vi "Acquire.vi"(8 "error in (no error)":errorcluster, 10 "Message Queues":T1, 11 "Hardware Resources in":T4) -> (0 "error out":errorcluster, 2 "Message Queues out":T1, 3 "Hardware Resources out":T4)   [LabVIEW 2019, in "Acquisition.lvlib"]
doc: "Perform the acquisition. Replace the contents of this diagram with calls to acquisition hardware."
uses:
  Acquisition.lvlib
  Hardware Configuration.ctl
  Signal Type.ctl
  Support/Message Queue/All Message Queues.ctl
  Support/Message Queue/Message Cluster.ctl
  Controls/Data Queue.ctl
  Controls/Acquired Data.ctl
  Controls/Data Notifier.ctl
  Support/Message Queue/Message Queue.lvlib
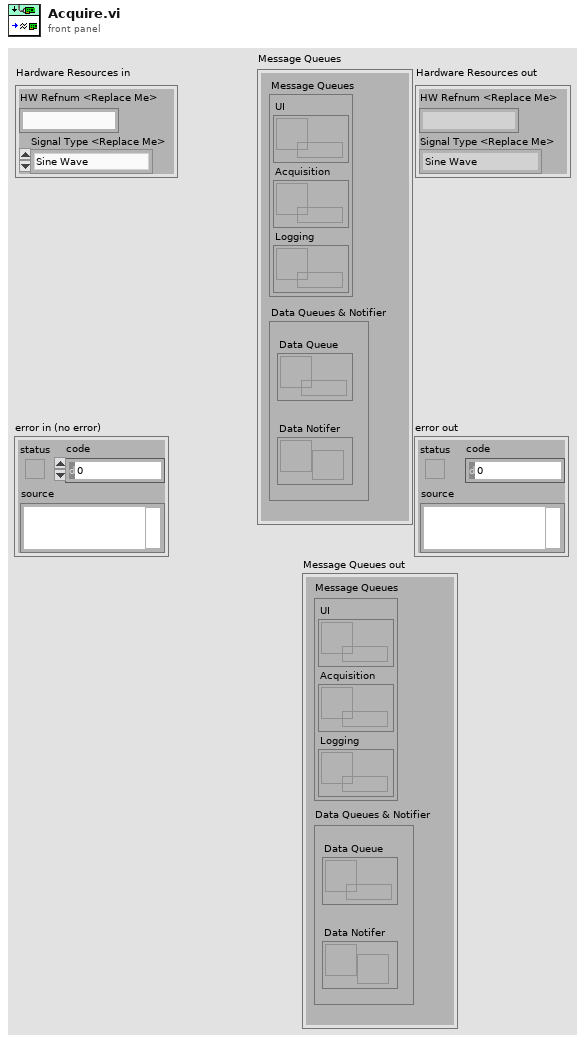
[diagram p1: front panel]
types:
  T1 = typedef "Message Queue.lvlib/All Message Queues.ctl" = cluster{"Message Queues":cluster{"UI":refnum<queue>, "Acquisition":refnum<queue>, "Logging":refnum<queue>}, "Data Queues & Notifier":cluster{"Data Queue":T2, "Data Notifer":T3}}
  T2 = typedef "Data Queue.ctl" = refnum<queue>
  T3 = typedef "Data Notifier.ctl" = refnum<notifier>
  T4 = typedef "Acquisition.lvlib/Hardware Configuration.ctl" = cluster{"HW Refnum <Replace Me>":string, "Signal Type <Replace Me>":T5}
  T5 = typedef "Acquisition.lvlib/Signal Type.ctl" = enum16{"Sine Wave", "Square with Noise"}
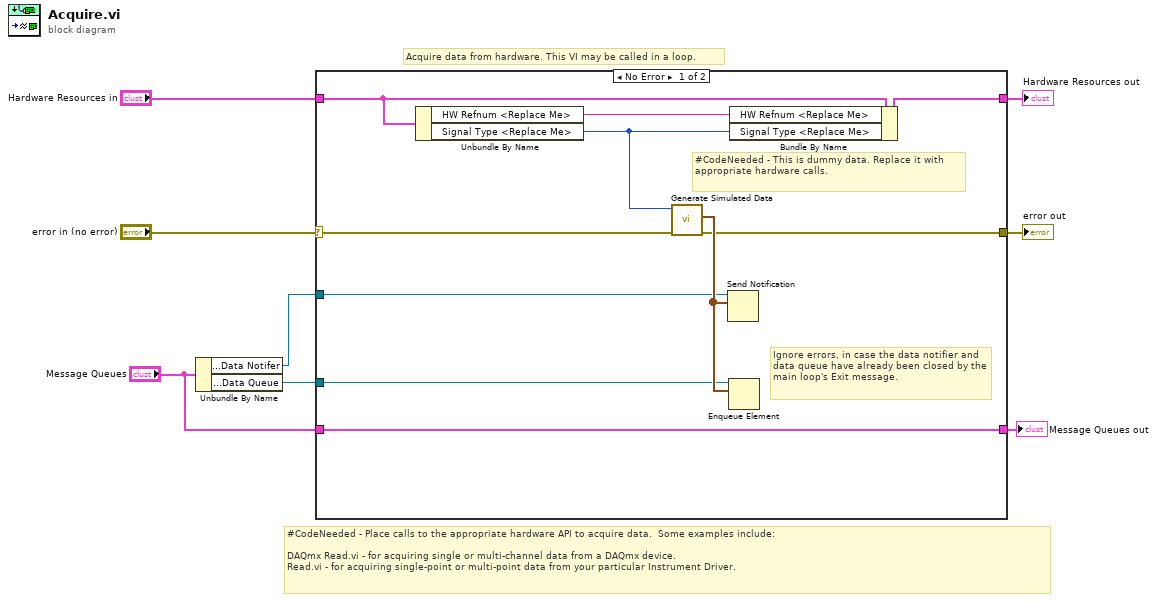
[diagram p0: block diagram]
diagram:
  # "Acquire data from hardware. This VI may be called in a loop."
  # "#CodeNeeded - Place calls to the appropriate hardware API to acquire data.  Some examples include:\n\nDAQmx Read.vi - for acquiring single or multi-channel data from a DAQmx device.\nRead.vi - for acquiring single-point or multi-point data from your particular Instrument Driver."
  n1 = Unbundle By Name("Message Queues") -> ("Data Queues & Notifier.Data Notifer"=w4:T3, "Data Queues & Notifier.Data Queue"=w3:T2)
  n2 = case shown="No Error" "error in (no error)" {
    selector: "error in (no error)" -> [w17 w20]
    tunnel: [w12 w20] -> w7
    tunnel: "Hardware Resources in" -> [w14 w21]
    tunnel: [w18 w21] -> w5
    tunnel: w4 -> [w11 _]
    tunnel: w3 -> [w10 _]
    tunnel: "Message Queues" -> [w9 w19]
    tunnel: [w9 w19] -> w1
    frame No Error {
      # "Ignore errors, in case the data notifier and data queue have already been closed by the main loop's Exit message."
      # "#CodeNeeded - This is dummy data. Replace it with appropriate hardware calls."
      n3 = Unbundle By Name(w14) -> ("HW Refnum <Replace Me>"=w15:string, "Signal Type <Replace Me>"=w16:T5)
      n4 = call "Generate Simulated Data.vi"("error in (no error)"=w17, "Signal Type"=w16) -> ("error out"=w12:errorcluster, "Graph Data"=w13:waveform(dbl)[])  [unwired: 8 in]
      n5 = Send Notification(notification=w13, notifier=w11) -> ()  [unwired: 1 in, 2 out]
      n6 = Enqueue Element(queue=w10, element=w13) -> ()  [unwired: 2 in, 3 out]
      n7 = Bundle By Name(cluster=w14, "HW Refnum <Replace Me>"=w15, "Signal Type <Replace Me>"=w16) -> (w18:T4)
    }
    frame Error {
    }
  }
  "Hardware Resources out" <- w5
  "error out" <- w7
  "Message Queues out" <- w1
